vi "tdms.vi"   [LabVIEW 2025]
uses:
  <vilib>/Utility/TDMS File Viewer/NI_TDMS File Viewer.lvlib
types:
  T1 = enum16{"open", "open or create", "create or replace", "create", "open (read-only)"}
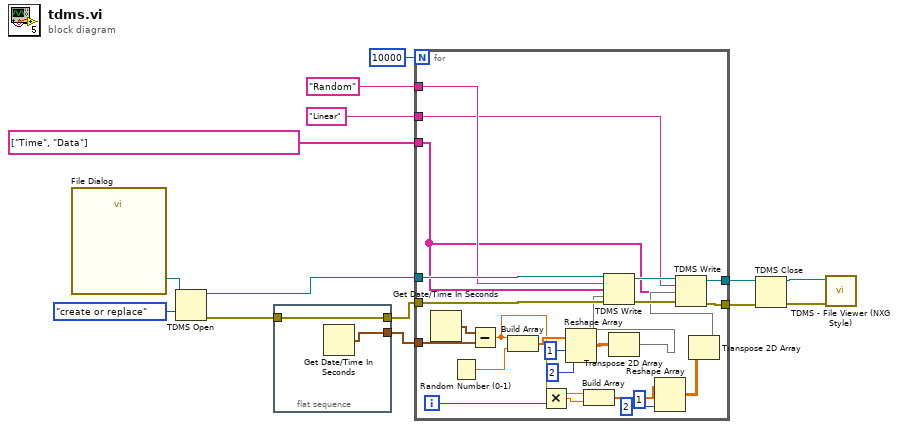
[diagram p0: block diagram]
diagram:
  n1 = call "File Dialog"() -> ("selected path"=w3:path)  [unwired: 12 in, 3 out]
  n2 = TDMS Open(10:T1."create or replace" ("operation (0:open)"), 11:w3) -> (0:w2:errorcluster, 3:w13:refnum<k34>)  [unwired: 5 in]
  n3 = flat-sequence {
    tunnel: [w16] -> w5
    tunnel: w2 -> [w15]
    tunnel: [w15] -> w1
    frame #0 {
      n4 = Get Date/Time In Seconds() -> (seconds since 1Jan1904=w16:timestamp)
    }
  }
  n5 = for {
    N: 10000 -> [_]
    tunnel: w13 -> [w41]
    tunnel: "Random" ("group name in (Untitled)") -> [w39]
    tunnel: "Linear" ("group name in (Untitled)") -> [w38]
    tunnel: string[] ["Time", "Data"] ("channel name(s) in (Untitled)") -> [w17]
    tunnel: w1 -> [w37]
    tunnel: [w35] -> w9
    tunnel: [w34] -> w8
    tunnel: w5 -> [w32]
    i -> [w30]
    n6 = Get Date/Time In Seconds() -> (seconds since 1Jan1904=w33:timestamp)
    n7 = Random Number (0-1)() -> (number: 0 to 1=w31:dbl)
    n8 = Subtract(x=w33, y=w32) -> (x-y=w24:dbl)
    n9 = Build Array(w24, w31) -> (w29:dbl[])
    n10 = Multiply(x=w24, y=w30) -> (x*y=w23:dbl)
    n11 = Reshape Array(w29, 1 ("dimension size"), 2 ("dimension size")) -> (w26:dbl[][])
    n12 = Build Array(w24, w23) -> (w22:dbl[])
    n13 = Transpose 2D Array(2D array=w26) -> (transposed array=w25:dbl[][])
    n14 = TDMS Write(0:w41, 5:w39, 7:w17, 9:w25, 11:w37) -> (4:w40:refnum<k34>, 15:w36:errorcluster)  [unwired: 1 in, 2 out]
    n15 = Reshape Array(w22, 1 ("dimension size"), 2 ("dimension size")) -> (w19:dbl[][])
    n16 = Transpose 2D Array(2D array=w19) -> (transposed array=w18:dbl[][])
    n17 = TDMS Write(0:w40, 5:w38, 7:w17, 9:w18, 11:w36) -> (4:w34:refnum<k34>, 15:w35:errorcluster)  [unwired: 1 in, 2 out]
  }
  n18 = TDMS Close(8:w9, 11:w8) -> (0:w7:errorcluster, 3:w6:path)
  n19 = call <vilib>:"TDMS - File Viewer (NXG Style).vi"("error in"=w7, "file in"=w6) -> ()  [unwired: 8 in, 2 out]
